vi "joe_read_output.vi"(4 "read and set output":T1={"mode"=0, "load"=FALSE, "inversion"=FALSE, "amplitude"=1.0, "offset"=0.0} {"offset" min=-3.0 max=4.0 format="%.2f"; "amplitude" min=-3.0 max=4.0 format="%.2f"; "mode" items=["TTL", "NIM", "ECL", "VAR"]}, 9 "output":u16(ring) items=["T0", "A", "B", "AB", "C", "D", "CD"], 11 "error in":errorcluster, 14 "read":bool) -> (15 "error out":errorcluster)   [LabVIEW 2011]
doc: "This VI is an example of how to use the DG535 subVIs programmatically .\nThe DG535 TRIGGER.VI sets the trigger mode , internal/burst trigger rate , burst count , burst period , external threshold voltage , external trigger slope and impedance of the DG535 .\nErrors are reported if the trigger rate is too high or if the burst period is out-of-range .\nThe DG535 DELAY.VI sets the delay time of channel i to t seconds relative to channel j . A \"Delay Linkage Error\" is caused by an attempt to totally disconnect a time reference from T0 . A \"Delay Range Error\" is reported when the total time delay for a channel exceeds 999.999999999995 seconds .\nDG535 SET OUTPUT.VI sets the mode , load , output polarity, amplitude and offset of the OUTPUT BNC selected while the DG535 READ OUTPUT.VI reads and displays these values ."
panel:
  out "decimal integer string 2":string
  in  "VISA resource":refnum<visa-resource-name>
  # "DG535 FOUR CHANNEL DIGITAL DELAY/PULSE GENERATOR"
  # "50 Ohm\nHigh Z"
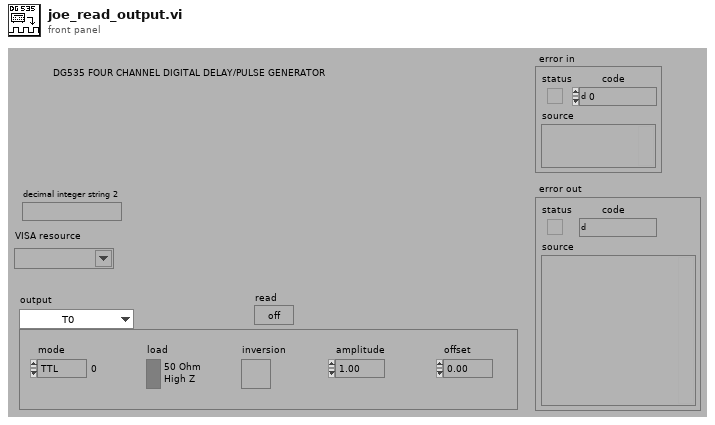
[diagram p1: front panel]
types:
  T1 = cluster{"mode":i32, "load":bool, "inversion":bool, "amplitude":dbl, "offset":dbl}
  T2 = cluster{"mode":u8, "load":bool, "inversion":bool, "amplitude":dbl, "offset":dbl}
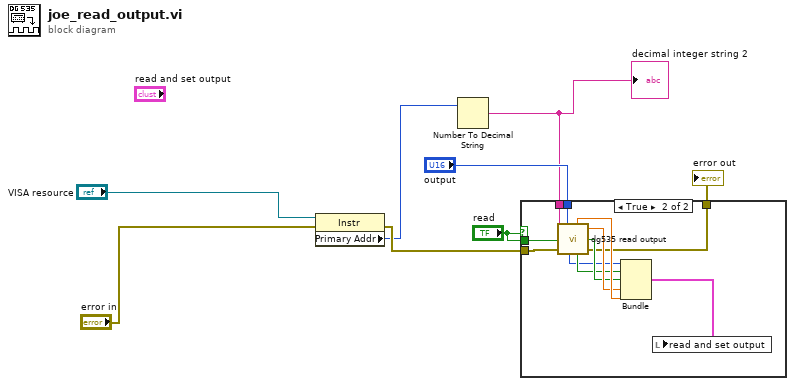
[diagram p0: block diagram]
diagram:
  n1 = property class="Instr"(reference="VISA resource", error in="error in") -> (error out=w3:errorcluster, "Primary Addr"=w2:u16)  [unwired: 1 in]
  n2 = Number To Decimal String(number=w2) -> (decimal integer string=w1:string)  [unwired: 1 in]
  "decimal integer string 2" <- w1
  n3 = case shown="True" "read" {
    tunnel: [w9 w15] -> w8
    tunnel: "read" -> [_ w14]
    tunnel: "output" -> [_ w13]
    tunnel: w1 -> [_ w12]
    tunnel: w3 -> [w9 w10]
    frame False {
    }
    frame True {
      n4 = call "dg535 read output.vi"("GPIB address"=w12, "output"=w13, "read"=w14, "error in"=w10) -> ("mode"=w11:u8, "offset"=w19:dbl, "amplitude"=w18:dbl, "inversion"=w17:bool, "load"=w16:bool, "error out"=w15:errorcluster)
      n5 = Bundle("mode"=w11, "load"=w16, "inversion"=w17, "amplitude"=w18, "offset"=w19) -> (w20:T2)  [unwired: 1 in]
      n6 = local write "read and set output"(w20) -> ()
    }
  }
  "error out" <- w8
